vi "Launcher - cRIO NI 9205 Demo.vi"(6 "Worker Alias":string="cRIO NI 9205 Demo", 8 "error in":errorcluster, 9 "Initialization Data":T1={"Client Name"="cRIO NI 9205 Demo", "Server IP Address"="", "Server Port"=9123, "Debugging Mode?"=FALSE}, 11 "cRIO NI 9205 Demo in":refnum<class "cRIO NI 9205 Demo.lvclass">) -> (0 "error out":errorcluster)   [LabVIEW 2017]
doc: "This VI launches the Head Worker of a Workers application."
uses:
  Workers/cRIO NI 9205 Demo/Initialization Data.ctl
  Workers/cRIO NI 9205 Demo/cRIO NI 9205 Demo.lvclass
  C:/Program Files (x86)/National Instruments/LabVIEW 2017/vi.lib/addons/_Workers/Library/Classes/Worker/Worker.lvclass
  <vilib>/addons/_Workers/Debugger/Debug Client/Debug Client.lvlib
panel:
  # "<- Change here the IP address of the Host PC"
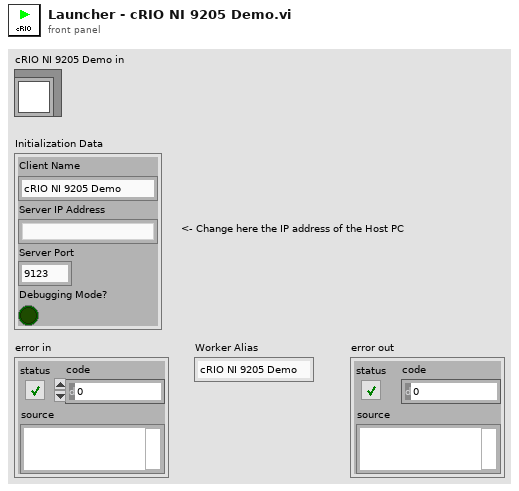
[diagram p1: front panel]
types:
  T1 = typedef "cRIO NI 9205 Demo.lvclass/Initialization Data.ctl" = cluster{"Client Name":string, "Server IP Address":string, "Server Port":u16, "Debugging Mode?":bool}
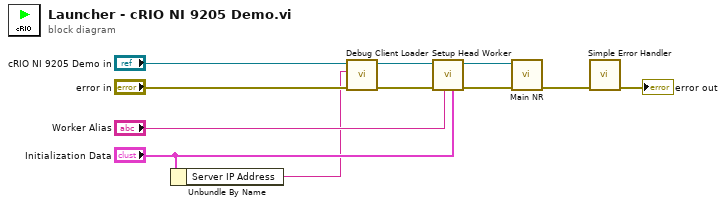
[diagram p0: block diagram]
diagram:
  n1 = Unbundle By Name("Initialization Data") -> ("Server IP Address"=w1:string)
  n2 = call <vilib>:"Debug Client Loader.vi"("error in (no error)"="error in", "Debug Server IP Address (127.0.0.1)"=w1, "Worker_"="cRIO NI 9205 Demo in") -> ("error out"=w5:errorcluster, "Worker_out"=w3:refnum<class "cRIO NI 9205 Demo.lvclass">)  [unwired: 7 in]
  n3 = call-dynamic "Setup Head Worker.vi"("Initalization Data"="Initialization Data", "Worker Alias"="Worker Alias", "error in"=w5, "Worker_"=w3) -> ("error out"=w11:errorcluster, "Worker_out"=w8:refnum<class "cRIO NI 9205 Demo.lvclass">)  [unwired: 6 in]
  n4 = call-dynamic "Main NR.vi"("error in"=w11, "cRIO NI 9205 Demo in"=w8) -> ("error out"=w9:errorcluster)  [unwired: 8 in, 1 out]
  n5 = call <vilib>:"Simple Error Handler.vi"("error in (no error)"=w9) -> ("error out"=→"error out":errorcluster)  [unwired: 4 in, 4 out]
